vi "Data Read.vi"(0 "VISA resource name":refnum<visa-resource-name>, 5 "error in (no error)":errorcluster) -> (14 "VISA resource name out":refnum<visa-resource-name>, 15 "Primary":dbl format="%#_6e", 17 "Secondary":dbl, 19 "error out":errorcluster)   [LabVIEW 2020, in "Keithley 2100 Series.lvlib"]
doc: "This VI reads a measurement or calculation from the instrument. It also returns the channel number and units of the measurement (if applicable).\nPrimary - Primary display reading\nSecondary - 2nd Function measurement."
uses:
  Keithley 2100 Series.lvlib
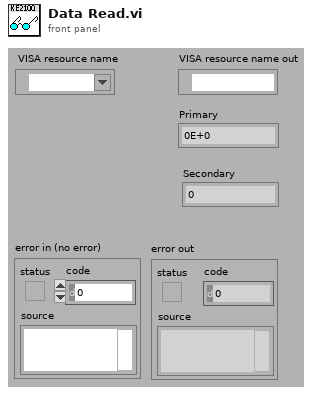
[diagram p1: front panel]
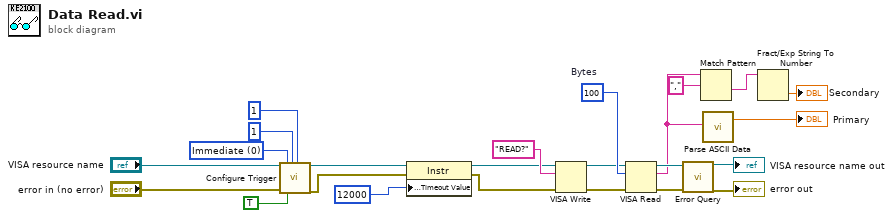
[diagram p0: block diagram]
diagram:
  w14 = u16 0 items=["Immediate", "Bus", "External"] ("Source (0: Immediate)")
  w24 = u32 100  # Bytes
  n1 = call "Configure Trigger.vi"("VISA resource name"="VISA resource name", "error in (no error)"="error in (no error)", "Source (0: Immediate)"=w14, "Auto Delay? (T: Auto)"=TRUE, "Sample Count (1)"=1, "Trigger Count (1)"=1 ("Sample Count (1)")) -> ("VISA resource name out"=w9:refnum<visa-resource-name>, "error out"=w8:errorcluster)  [unwired: 12 in]
  n2 = property class="Instr"(reference=w9, error in=w8, "General Settings:Timeout Value"=u32 12000) -> (reference out=w6:refnum<visa-resource-name>, error out=w7:errorcluster)
  n3 = VISA Write(VISA resource name=w6, write buffer="READ?", error in (no error)=w7) -> (VISA resource name out=w11:refnum<visa-resource-name>, error out=w10:errorcluster)  [unwired: 1 out]
  n4 = VISA Read(VISA resource name=w11, byte count=w24, error in (no error)=w10) -> (VISA resource name out=w23:refnum<visa-resource-name>, read buffer=w4:string, error out=w22:errorcluster)  [unwired: 1 out]
  n5 = call "Error Query.vi"("VISA resource name"=w23, "error in (no error)"=w22) -> ("VISA resource name out"=→"VISA resource name out":refnum<visa-resource-name>, "error out"=→"error out":errorcluster)  [unwired: 14 in, 2 out]
  n6 = Match Pattern(string=w4, regular expression=",") -> (after substring=w2:string)  [unwired: 1 in, 3 out]
  n7 = call "Parse ASCII Data.vi"("ASCII Data (Empty)"=w4) -> ("Measurement"=→"Primary":dbl)  [unwired: 18 in]
  n8 = Fract/Exp String To Number(string=w2) -> (number=→"Secondary":dbl)  [unwired: 3 in, 1 out]
